vi "Configure Frequency Range Scan.vi"(6 "step, Hz":u32, 8 "error in (no error)":errorcluster, 9 "stop, Hz":u32, 10 "start, Hz":u32, 11 "VI Probe in":refnum<class "PL MKS VI Probe.lvclass">) -> (0 "error out":errorcluster, 3 "VI Probe out":refnum<class "PL MKS VI Probe.lvclass">)   [LabVIEW 2015, in "PL MKS VI Probe.lvclass"]
doc: "Configures frequency scan, specified by start, stop and step frequency."
uses:
  PL MKS VI Probe.lvclass
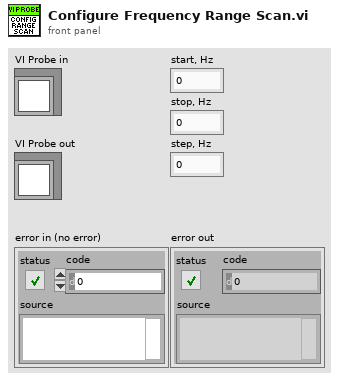
[diagram p1: front panel]
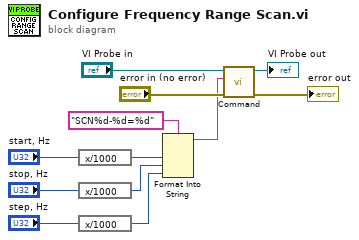
[diagram p0: block diagram]
diagram:
  n1 = expression code="x/1000"("start, Hz") -> (w3:u32)
  n2 = expression code="x/1000"("stop, Hz") -> (w2:u32)
  n3 = expression code="x/1000"("step, Hz") -> (w1:u32)
  n4 = Format Into String(format string="SCN%d-%d=%d", w3, w2, w1) -> (resulting string=w7:string)  [unwired: 2 in, 1 out]
  n5 = call "Command.vi"("error in (no error)"="error in (no error)", "command"=w7, "VI Probe in"="VI Probe in") -> ("error out"=→"error out":errorcluster, "VI Probe out"=→"VI Probe out":refnum<class "PL MKS VI Probe.lvclass">)  [unwired: 6 in, 1 out]
